vi "Custom Error Handler.vi"(8 "error in (no error)":errorcluster={"status"=TRUE, "code"=122, "source"="yo yo!"}) -> (0 "error out":errorcluster)   [LabVIEW 2013]
uses:
  <vilib>/Utility/file.llb/Read From Spreadsheet File (string).vi
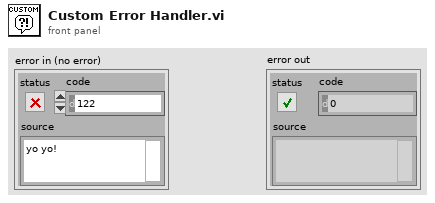
[diagram p1: front panel]
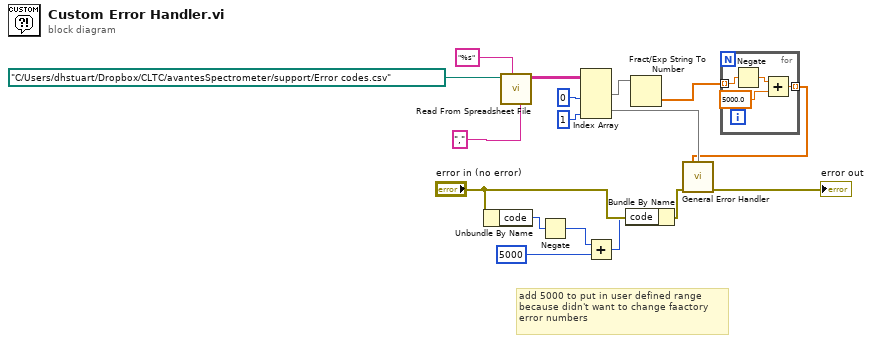
[diagram p0: block diagram]
diagram:
  # "add 5000 to put in user defined range\nbecause didn't want to change faactory\nerror numbers"
  n1 = Unbundle By Name("error in (no error)") -> ("code"=w2:i32)
  n2 = call-poly <vilib>:"Read From Spreadsheet File.vi"("delimiter (\\t)"="," ("delimiter (\\t)"), "format (%s)"="%s" ("format (%.3f)"), "file path (dialog if empty)"=path "C:/Users/dhstuart/Dropbox/CLTC/avantesSpectrometer/support/Error codes.csv") -> ("all rows"=w13:string[][])  [unwired: 4 in, 4 out]
  n3 = Negate(x=w2) -> (-x=w1:i32)
  n4 = Index Array(array=w13, index (col) #1=0 ("disabled index (col)"), index (col) #2=1 ("index (col)")) -> (element #1=w10:string[], element #2=w9:string[])  [unwired: 2 in]
  n5 = Add(x=w1, y=5000) -> (x+y=w6:i32)
  n6 = Bundle By Name(cluster="error in (no error)", "code"=w6) -> (w7:errorcluster)
  n7 = Fract/Exp String To Number(string=w10) -> (number=w5:dbl[])  [unwired: 3 in, 1 out]
  n8 = for {
    tunnel: w5 -> [w18] mode=indexing
    tunnel: [w20] -> w4 mode=indexing
    n9 = Negate(x=w18) -> (-x=w19:dbl)
    n10 = Add(x=w19, y=5000.0) -> (x+y=w20:dbl)
  }
  n11 = call <vilib>:"General Error Handler.vi"("[user-defined codes]"=w4, "[user-defined descriptions]"=w9, "error in (no error)"=w7) -> ("error out"=→"error out":errorcluster)  [unwired: 8 in, 4 out]
